vi "总磷氨氮版本号读取.vi"() -> (3 "固件版本号":string)   [LabVIEW 2016, in "氨氮.lvlib"]
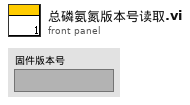
[diagram p1: front panel]
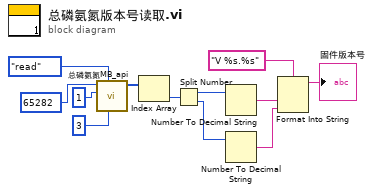
[diagram p0: block diagram]
diagram:
  n1 = call "总磷氨氮MB_api.vi"("Slave ID"=u8 3, "STEP"=enum16{"open", "read", "write", "close"}."read", "quantity"=u16 1, "starting address"=u16 65282) -> ("Registers"=w8:u16[])  [unwired: 5 in, 2 out]
  n2 = Index Array(array=w8) -> (element=w7:u16)  [unwired: 1 in]
  n3 = Split Number(x=w7) -> (hi(x)=w6:u8, lo(x)=w5:u8)
  n4 = Number To Decimal String(number=w6) -> (decimal integer string=w4:string)  [unwired: 1 in]
  n5 = Number To Decimal String(number=w5) -> (decimal integer string=w3:string)  [unwired: 1 in]
  n6 = Format Into String(format string="V %s.%s" ("格式字符串"), w4, w3) -> (resulting string=→"固件版本号":string)  [unwired: 2 in, 1 out]
